vi "Bus Interface.vi"(0 "AO":refnum<class "Analog Output.lvclass">, 1 "abort":bool, 5 "instruction":T2, 9 "input valid":bool) -> (6 "response":T1, 10 "done":bool, 14 "ready for input":bool)   [LabVIEW 2017, in "Analog IO.lvlib" / "Analog Output.lvclass"]
uses:
  Analog Output.lvclass
  <instrlib>/_niInstr/Instruction Framework/v1/FPGA/Interfaces/Address Space/Address Space Instruction.ctl
  <instrlib>/_niInstr/Instruction Framework/v1/FPGA/Typedefs/Response.ctl
  <instrlib>/_niInstr/Instruction Framework/v1/FPGA/Typedefs/niInstr Instruction Framework v1 FPGA.lvlib
  <instrlib>/_niInstr/Instruction Framework/v1/FPGA/Interfaces/Address Space/Address Space.lvclass
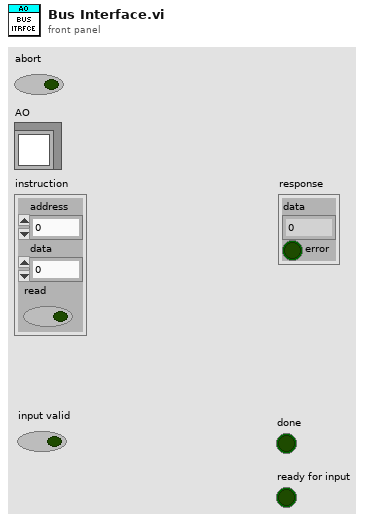
[diagram p1: front panel]
types:
  T1 = typedef "niInstr Instruction Framework v1 FPGA.lvlib/Response.ctl" = cluster{"data":u64, "error":bool}
  T2 = typedef "niInstr Instruction Framework Interfaces v1 FPGA.lvlib/Address Space.lvclass/Address Space Instruction.ctl" = cluster{"address":u32, "data":u64, "read":bool}
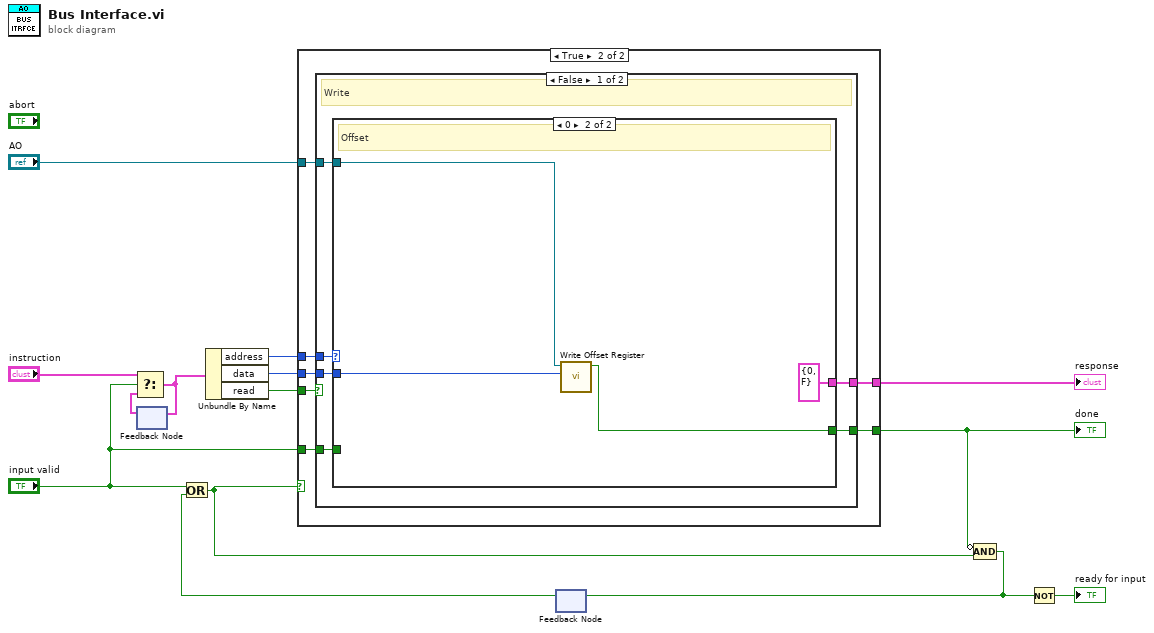
[diagram p0: block diagram]
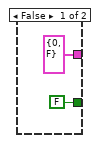
[diagram p2: hidden frame]
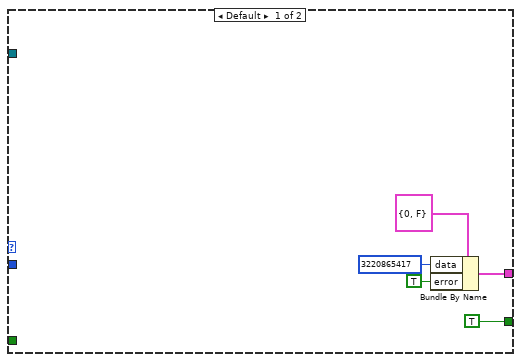
[diagram p3: hidden frame]
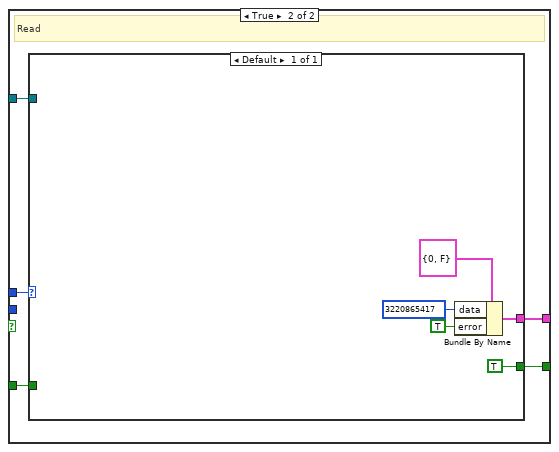
[diagram p4: hidden frame]
diagram:
  n1 = feedback #1() -> (w13:T2)  [unwired: 1 in]
  n2 = Select(t="instruction", s="input valid", f=w13) -> (s? t:f=w12:T2)
  n3 = feedback-in #1(w12) -> ()
  n4 = Unbundle By Name(w12) -> ("address"=w9:u32, "data"=w10:u64, "read"=w11:bool)
  n5 = feedback #2() -> (w3:bool)  [unwired: 1 in]
  n6 = Or(x="input valid", y=w3) -> (x .or. y?=w4:bool)
  n7 = case shown="True" w4 {
    tunnel: w11 -> [_ w23]
    tunnel: w9 -> [_ w22]
    tunnel: w10 -> [_ w21]
    tunnel: [T1 {"data"=0, "error"=FALSE} ("response") w20] -> w8
    tunnel: [FALSE ("Output Valid") w19] -> w1
    tunnel: "AO" -> [_ w18]
    tunnel: "input valid" -> [_ w17]
    frame False {
    }
    frame True {
      n8 = case shown="False" w23 {
        tunnel: w22 -> [w29 w43]
        tunnel: w21 -> [w28 _]
        tunnel: [w27 w42] -> w20
        tunnel: [w26 w41] -> w19
        tunnel: w18 -> [w25 w40]
        tunnel: w17 -> [w24 w39]
        frame False {
          # "Write"
          n9 = case shown="0" w29 {
            tunnel: w28 -> [_ w38]
            tunnel: [w31 T1 {"data"=0, "error"=FALSE} ("response")] -> w27
            tunnel: [TRUE ("done") w36] -> w26
            tunnel: w25 -> [_ w37]
            tunnel: w24 -> [_ _]
            frame Default {
              n10 = Bundle By Name(cluster=T1 {"data"=0, "error"=FALSE} ("response"), "data"=u64 3220865417, "error"=TRUE) -> (w31:T1)
            }
            frame 0 {
              # "Offset"
              n11 = call-dynamic "Write Offset Register.vi"("data"=w38, "AO in"=w37) -> ("done"=w36:bool)  [unwired: 9 in]
            }
          }
        }
        frame True {
          # "Read"
          n12 = case shown="Default" w43 {
            tunnel: [w45] -> w42
            tunnel: [TRUE ("done")] -> w41
            tunnel: w40 -> [_]
            tunnel: w39 -> [_]
            frame Default {
              n13 = Bundle By Name(cluster=T1 {"data"=0, "error"=FALSE} ("response"), "data"=u64 3220865417, "error"=TRUE) -> (w45:T1)
            }
          }
        }
      }
    }
  }
  "done" <- w1
  "response" <- w8
  n14 = Compound Arithmetic op=AND(invert w1, w4) -> (w5:bool)
  n15 = feedback-in #2(w5) -> ()
  n16 = Not(x=w5) -> (.not. x?=→"ready for input":bool)
